vi "Destruct.vi"(8 "error in (no error)":errorcluster) -> (0 "error out":errorcluster)   [LabVIEW 2018, in "Tag Engine.lvlib" / "Tag Core.lvclass"]
doc: "Destroy every Tag and then the Tag store"
uses:
  Tag Core.lvclass
  Tag Core.lvclass/Tag Core.ctl
  Tag/Tag.lvclass
  Tag/Tag.lvclass/Tag.ctl
  Tag/Read Name.vi
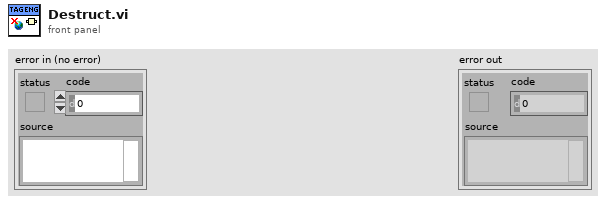
[diagram p1: front panel]
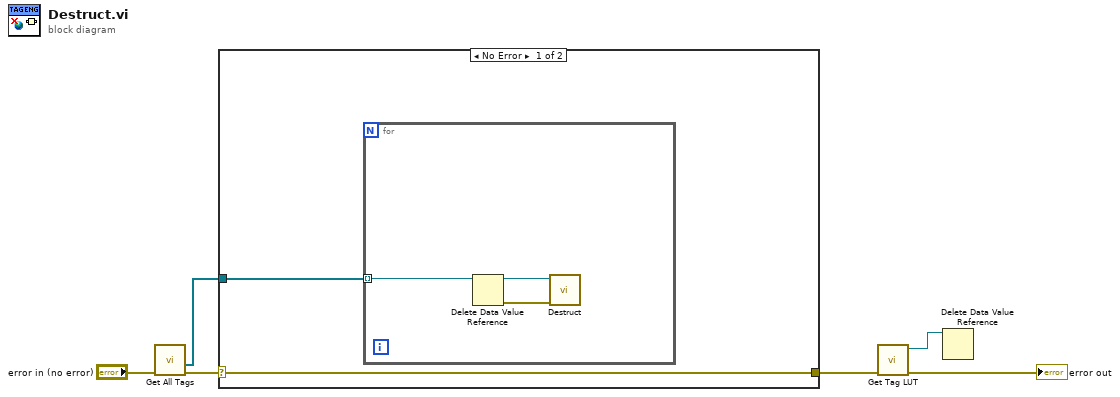
[diagram p0: block diagram]
diagram:
  n1 = call "Get All Tags.vi"("error in (no error)"="error in (no error)") -> ("error out"=w3:errorcluster, "Tag Refs"=w2:refnum<data-value>[])  [unwired: 8 in, 1 out]
  n2 = case shown="No Error" w3 {
    selector: w3 -> [w8 w12]
    tunnel: [w8 w12] -> w6
    tunnel: w2 -> [w7 _]
    frame No Error {
      n3 = for {
        tunnel: w7 -> [w11] mode=indexing
        n4 = Delete Data Value Reference(data value reference=w11) -> (data value=w10:refnum<class "Tag.lvclass">, error out=w9:errorcluster)  [unwired: 1 in]
        n5 = call "Destruct.vi"("error in (no error)"=w9, "Tag in"=w10) -> ()  [unwired: 9 in, 1 out]
      }
    }
    frame Error {
    }
  }
  n6 = call "Get Tag LUT.vi"("error in (no error)"=w6) -> ("error out"=→"error out":errorcluster, "Tag LUT Out"=w5:refnum<data-value>)  [unwired: 9 in]
  n7 = Delete Data Value Reference(data value reference=w5) -> ()  [unwired: 1 in, 2 out]
